vi "Main Page.vi"(8 "error in (no error)":errorcluster, 11 "Node Ptr":T1 format="%.0x") -> (0 "error out":errorcluster)   [LabVIEW 2015, in "Waveform-Processing-Custom-Device System Explorer.lvlib"]
uses:
  Waveform-Processing-Custom-Device System Explorer.lvlib
  <vilib>/NI Veristand/Custom Device API/Custom Device Item Ref.ctl
  Shared/Types/FG Action.ctl
  Types/UI Refs Ctl.ctl
  Shared/Constants.vi
  <vilib>/NI Veristand/Custom Device API/Set Item Property (Boolean).vi
  <vilib>/NI VeriStand/Custom Device API/Custom Device API.lvlib
  Shared/Waveform-Processing-Custom-Device Shared.lvlib
  Shared/Running Average/Running Average.lvlib
  Shared/Single Point/SinglePoint.lvlib
panel:
  in  "Header 2":cluster{"Section Name":string}={"Section Name"="Custom Device Item Settings"}
  out "Task Rate (Hz)":dbl
  in  "Buffer Length (s)":dbl format="%#_6f"
  out "Buffer Length (samples)":u32
  in  "Description":string
  in  "Remove Channel":bool
  in  "Add Channel":bool
  in  "Selected Waveforms":i32[](listbox)
  in  "Waveform Task":u16(ring) items=["Waveform1"=11, "Waveform2"=15]
  in  "Available Waveforms":i32[](listbox)
  in  "Single-point":bool
  in  "Running Average":bool
  in  "Header":cluster{"Section Name":string}={"Section Name"="Custom Device Item Settings"}
  in  "Name":string
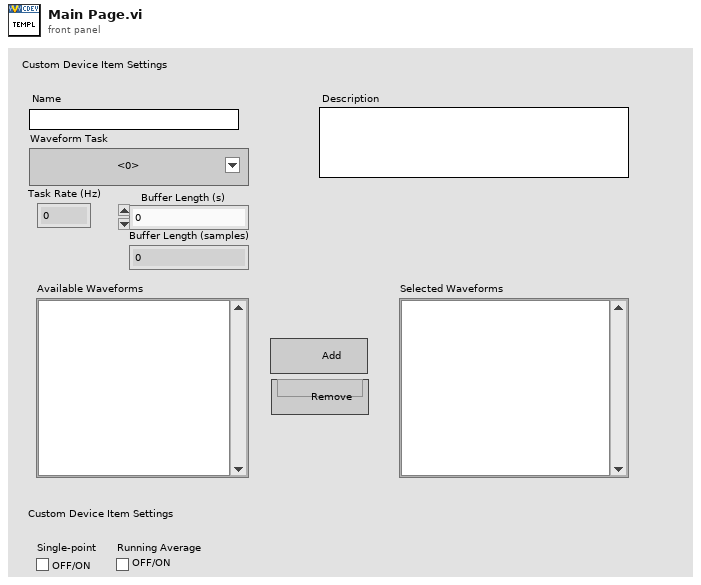
[diagram p1: front panel]
types:
  T1 = typedef "Custom Device API.lvlib/Custom Device Item Ref.ctl" = u64
  T2 = typedef "Waveform-Processing-Custom-Device Shared.lvlib/UI Refs Ctl.ctl" = cluster{"Selected Waveforms":refnum<vi>, "Available Waveforms":refnum<vi>, "Wfm Task Rate (Hz)":refnum<vi>, "Buffer Length (s)":refnum<vi>, "Buffer Length (samples)":refnum<vi>, "Add Channel":refnum<vi>, "Remove Channel":refnum<vi>, "Running Average":refnum<vi>, "Single-point":refnum<vi>, "Waveform Task":refnum<vi>}
  T3 = typedef "Waveform-Processing-Custom-Device Shared.lvlib/FG Action.ctl" = enum8{"GET", "SET"}
  T4 = typedef "Custom Device API.lvlib/Custom Device Item Info.ctl" = cluster{"Name":string, "Is Channel":bool, "GUID":string, "Is Waveform":bool}
  T5 = typedef "Waveform-Processing-Custom-Device Shared.lvlib/Custom Device Settings.ctl" = cluster{"CD Task Dependency":T1, "CD Task Dependency Ref":T1, "CD Task Available Wfms":string[], "CD Task Selected Wfms":string[], "Buffer Length (s)":dbl, "Buffer Length (samples)":u32, "Single-point Enabled":bool, "Running Average Enabled":bool, "Task Rate":dbl}
  T6 = typedef "Custom Device API.lvlib/Custom Device Commands.ctl" = enum16{"Default", "Item renamed", "Shutdown", "Dynamic button pressed"}
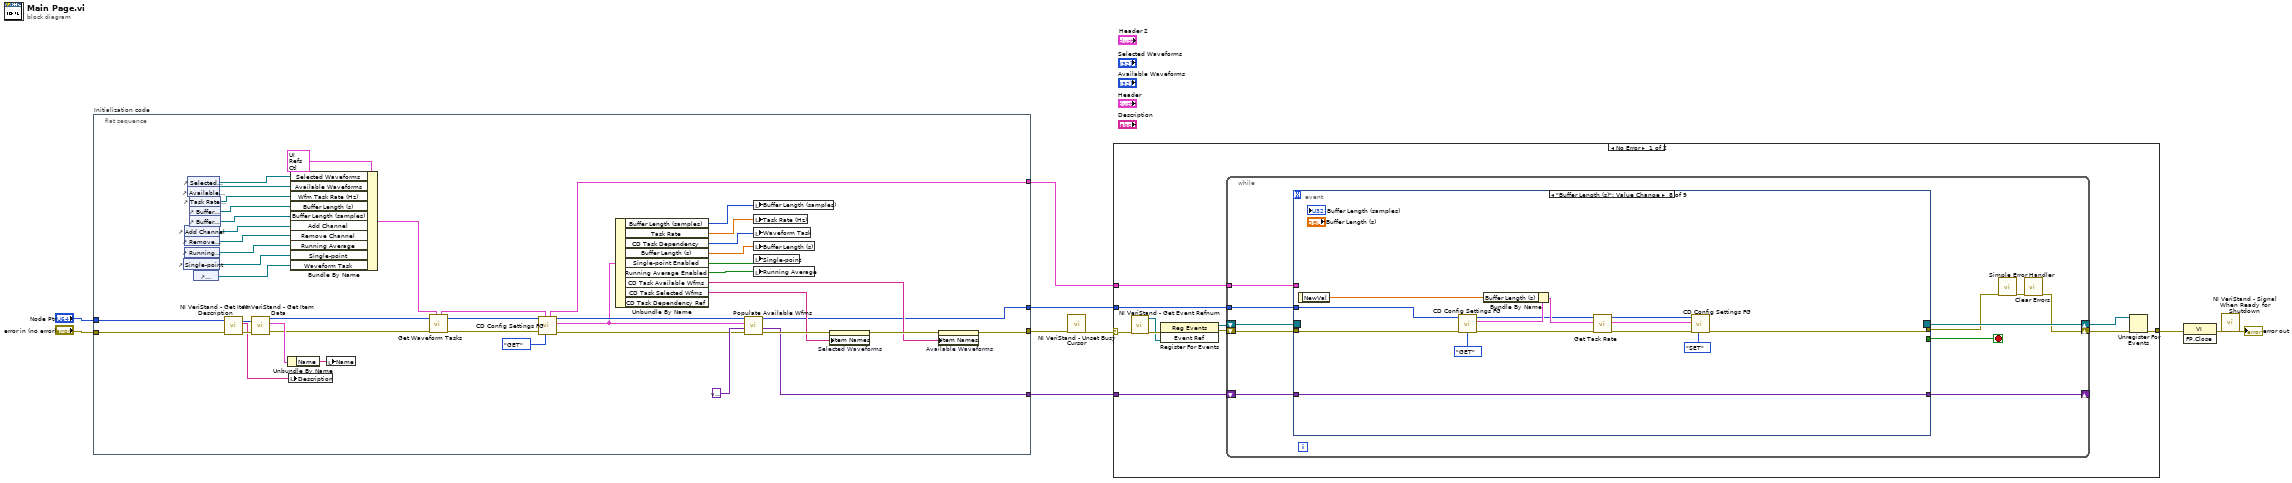
[diagram p0: block diagram]
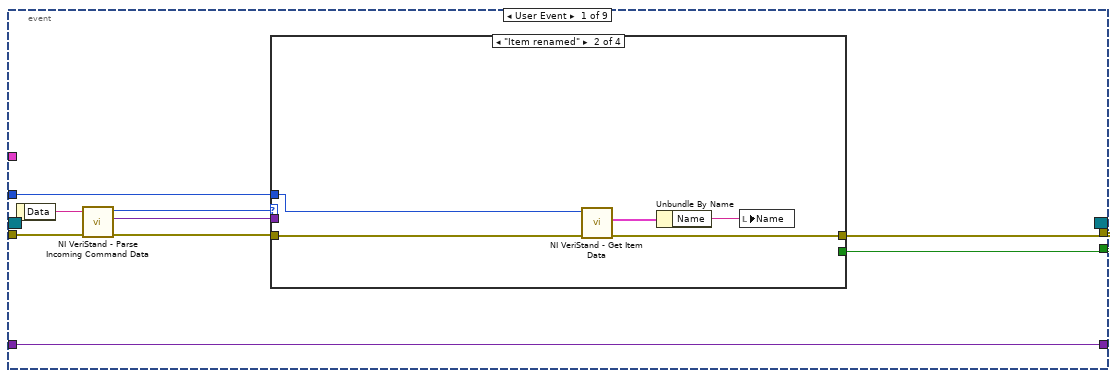
[diagram p2: hidden frame]
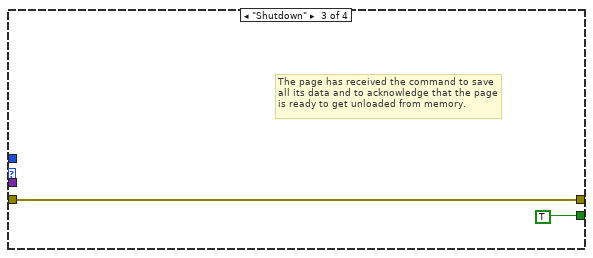
[diagram p4: hidden frame]
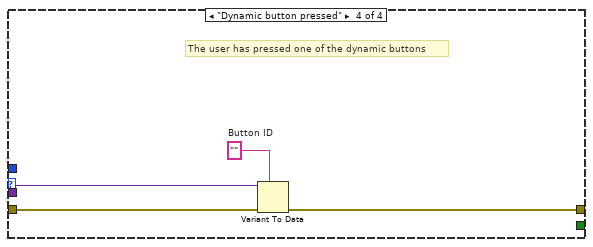
[diagram p5: hidden frame]
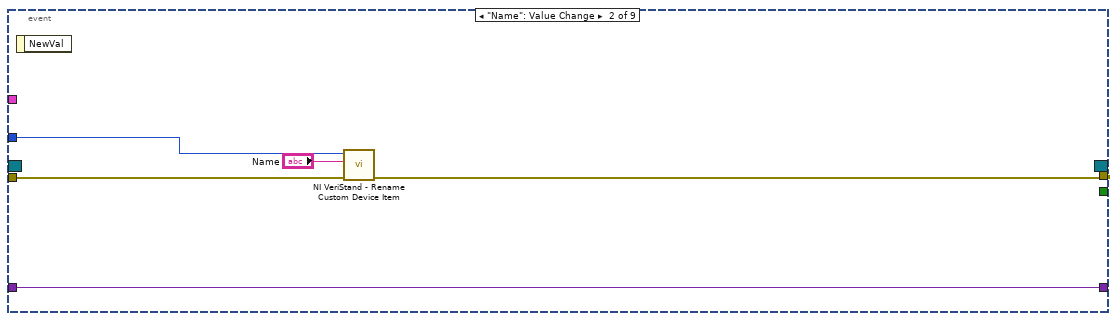
[diagram p6: hidden frame]
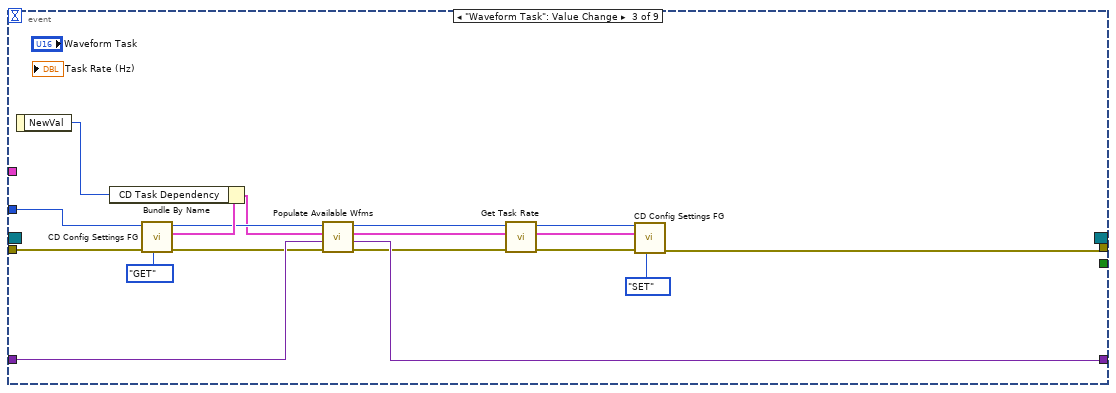
[diagram p7: hidden frame]
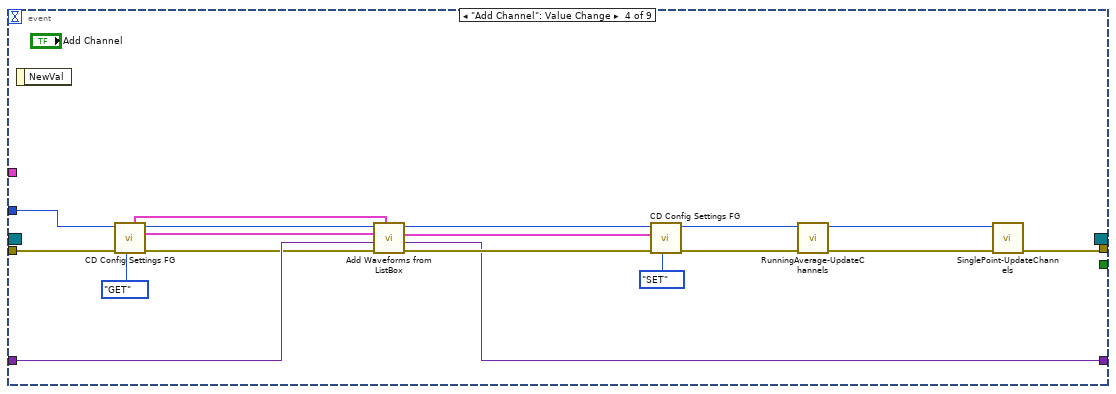
[diagram p8: hidden frame]
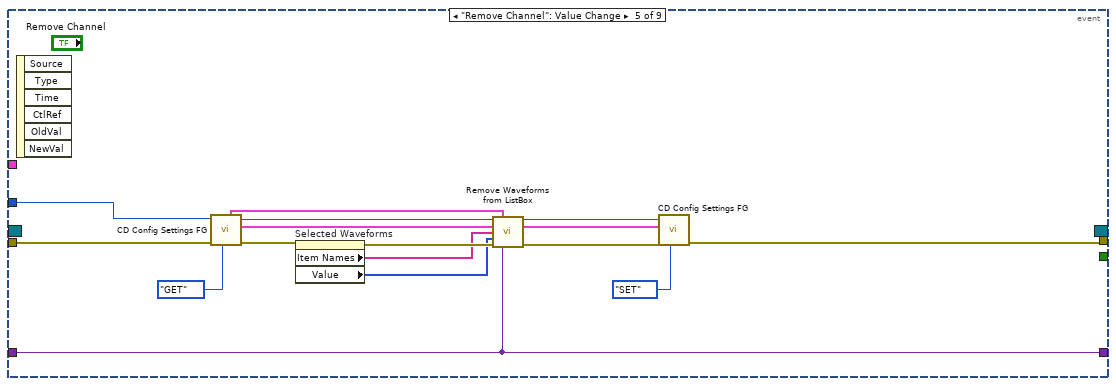
[diagram p9: hidden frame]
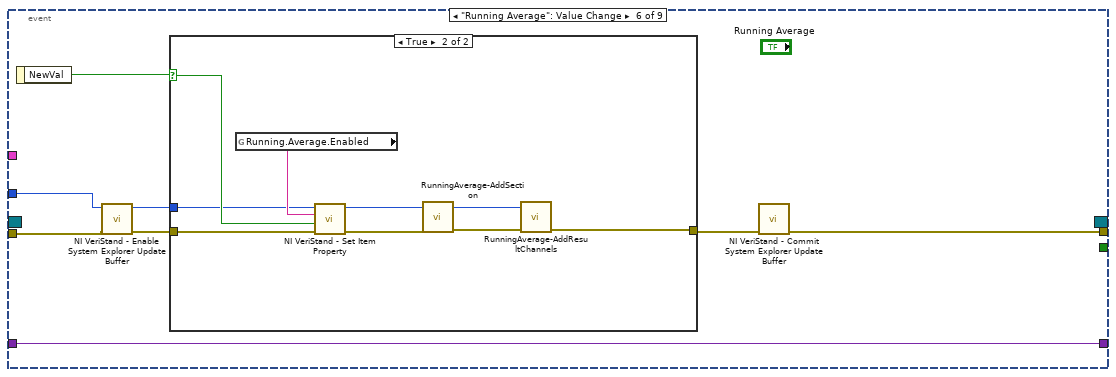
[diagram p10: hidden frame]
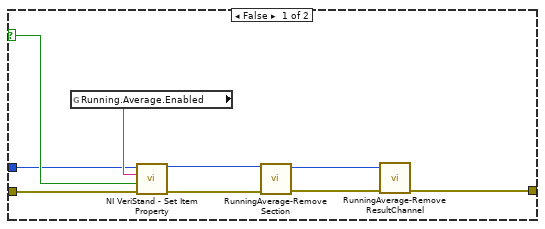
[diagram p11: hidden frame]
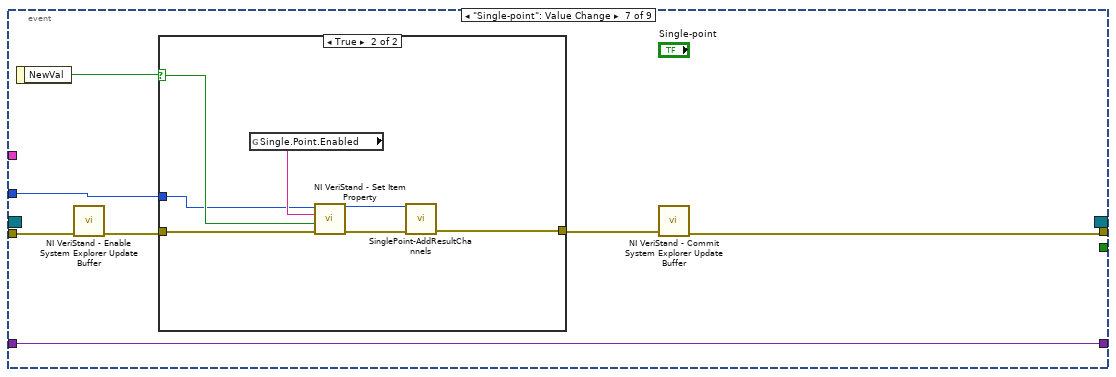
[diagram p12: hidden frame]
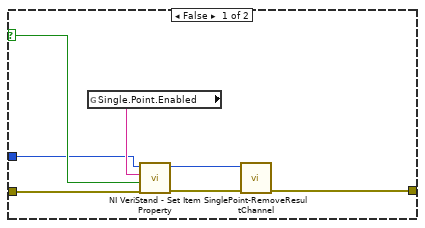
[diagram p13: hidden frame]
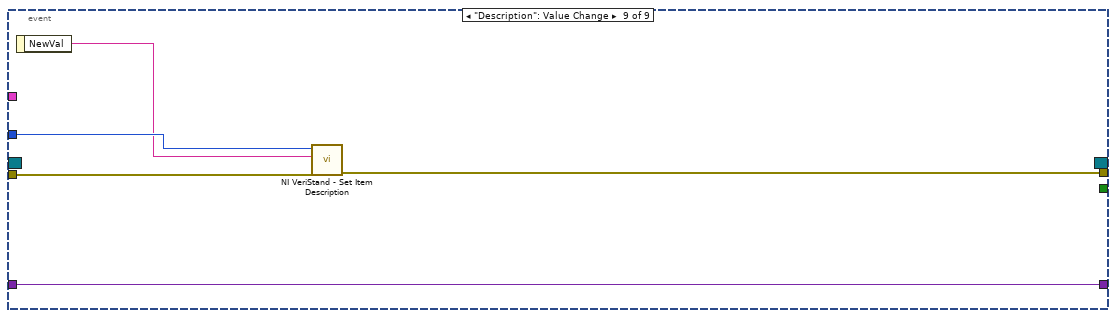
[diagram p14: hidden frame]
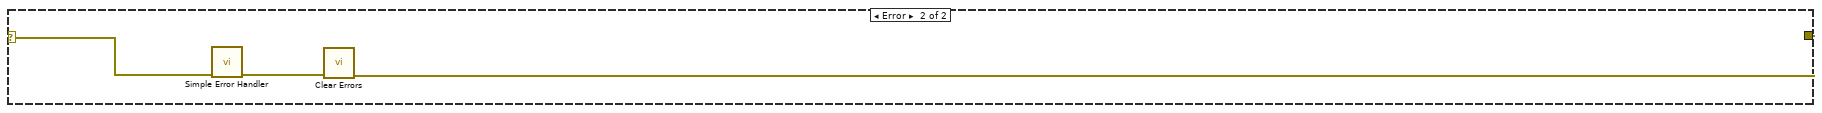
[diagram p15: hidden frame]
diagram:
  n1 = flat-sequence "Initialization code" {
    tunnel: "error in (no error)" -> [w52]
    tunnel: "Node Ptr" -> [w51]
    tunnel: [w38] -> w1
    tunnel: [w15] -> w4
    tunnel: [w13] -> w3
    tunnel: [w16] -> w2
    frame #0 {
      n2 = control-ref of="Single-point"() -> (w35:refnum<vi>)
      n3 = control-ref of="Add Channel"() -> (w32:refnum<vi>)
      n4 = control-ref of="Remove Channel"() -> (w33:refnum<vi>)
      n5 = control-ref of="Running Average"() -> (w34:refnum<vi>)
      n6 = control-ref of="Selected Waveforms"() -> (w27:refnum<vi>)
      n7 = control-ref of="Available Waveforms"() -> (w28:refnum<vi>)
      n8 = control-ref of="Task Rate (Hz)"() -> (w29:refnum<vi>)
      n9 = control-ref of="Buffer Length (s)"() -> (w30:refnum<vi>)
      n10 = control-ref of="Buffer Length (samples)"() -> (w31:refnum<vi>)
      n11 = control-ref of="Waveform Task"() -> (w17:refnum<vi>)
      n12 = call <vilib>:"NI VeriStand - Get Item Description.vi"("error in (no error)"=w52, "Item Ref in"=w51) -> ("error out"=w50:errorcluster, "Description"=w47:string, "Item Ref out"=w53:T1)  [unwired: 7 out]
      n13 = call <vilib>:"NI VeriStand - Get Item Data.vi"("error in (no error)"=w50, "Item Ref in"=w53) -> ("error out"=w24:errorcluster, "Item Info"=w49:T4, "Item Ref out"=w18:T1)  [unwired: 7 out]
      n14 = Unbundle By Name(w49) -> ("Name"=w48:string)
      n15 = local write "Description"(w47) -> ()
      n16 = Bundle By Name(cluster=T2 {"Selected Waveforms"=refnum, "Available Waveforms"=refnum, "Wfm Task Rate (Hz)"=refnum, "Buffer Length (s)"=refnum, "Buffer Length (samples)"=refnum, "Add Channel"=refnum, "Remove Channel"=refnum, "Running Average"=refnum, "Single-point"=refnum, "Waveform Task"=refnum} ("UI Refs"), "Selected Waveforms"=w27, "Available Waveforms"=w28, "Wfm Task Rate (Hz)"=w29, "Buffer Length (s)"=w30, "Buffer Length (samples)"=w31, "Add Channel"=w32, "Remove Channel"=w33, "Running Average"=w34, "Single-point"=w35, "Waveform Task"=w17) -> (w23:T2)
      n17 = local write "Name"(w48) -> ()
      n18 = call "Get Waveform Tasks.vi"("Custom Device ref in"=w18, "error in"=w24, "UI Refs in"=w23) -> ("UI Refs out"=w22:T2, "Custom Device ref out"=w21:T1, "error out"=w25:errorcluster)  [unwired: 5 in]
      n19 = call "CD Config Settings FG.vi"("Action"=FG_Action."GET", "UI Refs"=w22, "error in (no error)"=w25, "Item Ref"=w21) -> ("error out"=w20:errorcluster, "CD Settings out"=w11:T5, "Item Ref out"=w19:T1, "UI Refs out"=w16:T2)  [unwired: 4 in]
      n20 = Unbundle By Name(w11) -> ("Buffer Length (samples)"=w12:u32, "Task Rate"=w14:dbl, "CD Task Dependency"=w26:T1, "Buffer Length (s)"=w44:dbl, "Single-point Enabled"=w46:bool, "Running Average Enabled"=w45:bool, "CD Task Available Wfms"=w39:string[], "CD Task Selected Wfms"=w40:string[])  [unwired: 1 out]
      n21 = call "Populate Available Wfms.vi"("error in"=w20, "ListBox Variant"=variant, "CD Settings"=w11, "CustomDevice Ref"=w19) -> ("error out"=w42:errorcluster, "ListBox Variant"=w38:variant, "CustomDevice Ref"=w13:T1)  [unwired: 4 in, 1 out]
      n22 = local write "Buffer Length (samples)"(w12) -> ()
      n23 = local write "Task Rate (Hz)"(w14) -> ()
      n24 = local write "Waveform Task"(w26) -> ()
      n25 = local write "Buffer Length (s)"(w44) -> ()
      n26 = local write "Single-point"(w46) -> ()
      n27 = local write "Running Average"(w45) -> ()
      n28 = property on="Selected Waveforms" class="LstBox (strict)"(error in=w42, "Item Names"=w40) -> (error out=w41:errorcluster)  [unwired: 1 in, 1 out]
      n29 = property on="Available Waveforms" class="LstBox (strict)"(error in=w41, "Item Names"=w39) -> (error out=w15:errorcluster)  [unwired: 1 in, 1 out]
    }
  }
  n30 = call <vilib>:"NI VeriStand - Unset Busy Cursor.vi"("error in (no error)"=w4) -> ("error out"=w6:errorcluster)  [unwired: 10 out]
  n31 = case shown="No Error" w6 {
    selector: w6 -> [w57 w221]
    tunnel: [w61 w219] -> w10
    tunnel: w3 -> [w56 _]
    tunnel: w1 -> [w55 _]
    tunnel: w2 -> [w54 _]
    frame No Error {
      n32 = call <vilib>:"NI VeriStand - Get Event Refnum.vi"("error in (no error)"=w57) -> ("error out"=w64:errorcluster, "Event Ref"=w60:refnum<user-event>)  [unwired: 9 out]
      n33 = register-events(error in=w64, w60) -> (reference out=w58:refnum<event-registration>, error out=w59:errorcluster)  [unwired: 1 in]
      n34 = while {
        shift-right: [w71] -> w62
        shift-left: w59 -> [w67]
        shift-right: [w75] -> w63
        shift-left: w58 -> [w74]
        tunnel: w56 -> [w70]
        shift-right: [w69] -> _
        shift-left: w55 -> [w68]
        tunnel: w54 -> [w65]
        stop <- w73 stop-if-true
        n35 = event shown="[7] \"Buffer Length (s)\": Value Change" {
          selector: w74 -> [_ _ _ _ _ _ _ _ _]
          dyn-events: [_ _ _ _ _ _ _ _ _] -> w75
          timeout: _ -> [_ _ _ _ _ _ _ _ _]
          tunnel: w67 -> [w84 w101 w116 w131 w150 w157 w182 w212 w218]
          tunnel: [w80 _ _ _ _ _ _ _ _] -> w73
          tunnel: [w79 w100 w102 w126 w139 w154 w179 w200 w217] -> w66
          tunnel: w70 -> [w77 w98 w115 w137 w153 w159 w184 w210 w216]
          tunnel: [w76 w97 w119 w121 w138 w158 w183 w213 w214] -> w69
          tunnel: w68 -> [w76 w97 w118 w123 w138 w158 w183 w213 w214]
          tunnel: w65 -> [_ _ _ _ _ _ _ _ _]
          event User Event {
            n36 = event-data() -> ("Data"=w83:string)  [unwired: 1 out]
            n37 = call <vilib>:"NI VeriStand - Parse Incoming Command Data.vi"("error in (no error)"=w84, "Incoming data"=w83) -> ("error out"=w82:errorcluster, "Outgoing data"=w78:variant, "Action"=w81:T6)  [unwired: 7 out]
            n38 = case shown="\"Item renamed\"" w81 {
              tunnel: w82 -> [w85 w90 w91 w96]
              tunnel: [_ _ TRUE _] -> w80
              tunnel: [w85 w88 w91 w93] -> w79
              tunnel: w78 -> [_ _ _ w95]
              tunnel: w77 -> [_ w86 _ _]
              frame "Default", Default {
              }
              frame "Item renamed" {
                n39 = call <vilib>:"NI VeriStand - Get Item Data.vi"("error in (no error)"=w90, "Item Ref in"=w86) -> ("error out"=w88:errorcluster, "Item Info"=w89:T4)  [unwired: 8 out]
                n40 = Unbundle By Name(w89) -> ("Name"=w87:string)
                n41 = local write "Name"(w87) -> ()
              }
              frame "Shutdown" {
                # "The page has received the command to save all its data and to acknowledge that the page is ready to get unloaded from memory."
              }
              frame "Dynamic button pressed" {
                w94 = ""  # Button ID
                # "The user has pressed one of the dynamic buttons"
                n42 = Variant To Data(error in=w96, type=w94, Variant=w95) -> (error out=w93:errorcluster)  [unwired: 1 out]
              }
            }
          }
          event "Name": Value Change {
            n43 = event-data() -> ()  [unwired: 2 out]
            n44 = call <vilib>:"NI VeriStand - Rename Custom Device Item.vi"("error in (no error)"=w101, "New Name"="Name", "Item Ref in"=w98) -> ("error out"=w100:errorcluster)  [unwired: 1 in, 7 out]
          }
          event "Waveform Task": Value Change {
            n45 = event-data() -> ("NewVal"=w117:u16)  [unwired: 1 out]
            n46 = call "CD Config Settings FG.vi"("Action"=FG_Action."GET", "error in (no error)"=w116, "Item Ref"=w115) -> ("error out"=w111:errorcluster, "CD Settings out"=w114:T5, "Item Ref out"=w110:T1)  [unwired: 5 in, 1 out]
            n47 = Bundle By Name(cluster=w114, "CD Task Dependency"=w117) -> (w109:T5)
            n48 = call "Populate Available Wfms.vi"("error in"=w111, "ListBox Variant"=w118, "CD Settings"=w109, "CustomDevice Ref"=w110) -> ("error out"=w108:errorcluster, "ListBox Variant"=w119:variant, "CD Settings out"=w107:T5, "CustomDevice Ref"=w106:T1)  [unwired: 4 in]
            n49 = call "Get Task Rate.vi"("error in"=w108, "CD Settings"=w107, "CustomDevice Ref"=w106) -> ("error out"=w104:errorcluster, "CD Settings out"=w103:T5, "CustomDevice Ref out"=w105:T1)  [unwired: 6 in]
            n50 = call "CD Config Settings FG.vi"("Action"=FG_Action."SET", "error in (no error)"=w104, "CD Settings in"=w103, "Item Ref"=w105) -> ("error out"=w102:errorcluster)  [unwired: 4 in, 3 out]
          }
          event "Add Channel": Value Change {
            n51 = event-data() -> ()  [unwired: 2 out]
            n52 = call "CD Config Settings FG.vi"("Action"=FG_Action."GET", "error in (no error)"=w131, "Item Ref"=w137) -> ("error out"=w122:errorcluster, "CD Settings out"=w133:T5, "Item Ref out"=w130:T1, "UI Refs out"=w120:T2)  [unwired: 5 in]
            n53 = call "Add Waveforms from ListBox.vi"("UI Refs"=w120, "error in (no error)"=w122, "Wfm Ref LUT"=w123, "CD Settings in"=w133, "Custom Device Ref in"=w130) -> ("error out"=w136:errorcluster, "Wfm Ref LUT out"=w121:variant, "CD Settings out"=w132:T5, "Custom Device Ref out"=w129:T1)  [unwired: 1 in]
            n54 = call "CD Config Settings FG.vi"("Action"=FG_Action."SET", "error in (no error)"=w136, "CD Settings in"=w132, "Item Ref"=w129) -> ("error out"=w128:errorcluster, "Item Ref out"=w125:T1)  [unwired: 4 in, 2 out]
            n55 = call "RunningAverage-UpdateChannels.vi"("Error in"=w128, "Custom Device ref in"=w125) -> ("Error out"=w127:errorcluster, "Custom Device ref out"=w124:T1)  [unwired: 8 in]
            n56 = call "SinglePoint-UpdateChannels.vi"("Error in"=w127, "Custom Device ref in"=w124) -> ("Error out"=w126:errorcluster)  [unwired: 8 in, 1 out]
          }
          event "Remove Channel": Value Change {
            n57 = event-data() -> ()  [unwired: 7 out]
            n58 = call "CD Config Settings FG.vi"("Action"=FG_Action."GET", "error in (no error)"=w150, "Item Ref"=w153) -> ("error out"=w149:errorcluster, "CD Settings out"=w144:T5, "Item Ref out"=w143:T1, "UI Refs out"=w142:T2)  [unwired: 5 in]
            n59 = property on="Selected Waveforms" class="LstBox (strict)"(error in=w149) -> (error out=w148:errorcluster, "Item Names"=w145:string[], "Value"=w146:i32[])  [unwired: 1 in, 1 out]
            n60 = call "Remove Waveforms from ListBox.vi"("Custom Device Ref in"=w143, "UI Refs"=w142, "CD Settings in"=w144, "Item Names"=w145, "Value"=w146, "error in (no error)"=w148, "Waveform Ref LUT"=w138) -> ("Custom Device Ref out"=w141:T1, "CD Settings out"=w140:T5, "error out"=w147:errorcluster)  [unwired: 6 in]
            n61 = call "CD Config Settings FG.vi"("Action"=FG_Action."SET", "error in (no error)"=w147, "CD Settings in"=w140, "Item Ref"=w141) -> ("error out"=w139:errorcluster)  [unwired: 4 in, 3 out]
          }
          event "Running Average": Value Change {
            n62 = event-data() -> ("NewVal"=w160:bool)  [unwired: 1 out]
            n63 = call <vilib>:"NI VeriStand - Enable System Explorer Update Buffer.vi"("error in (no error)"=w157) -> ("error out"=w156:errorcluster)  [unwired: 10 in]
            n64 = case shown="True" w160 {
              selector: w160 -> [w167 w177]
              tunnel: w156 -> [w169 w170]
              tunnel: [w162 w171] -> w155
              tunnel: w159 -> [w166 w174]
              frame False {
                n65 = global read "Constants.vi" "Running.Average.Enabled"() -> (w168:string)
                n66 = call-poly <vilib>:"NI VeriStand - Set Item Property.vi"("error in (no error)"=w169, "Value"=w167, "Property Name"=w168, "Item Ref in"=w166) -> ("error out"=w164:errorcluster, "Item Ref out"=w165:T1)  [unwired: 5 in, 1 out]
                n67 = call "RunningAverage-RemoveSection.vi"("Error in"=w164, "Custom Device ref"=w165) -> ("Error out"=w163:errorcluster, "Custom Device ref out"=w161:T1)  [unwired: 8 in]
                n68 = call "RunningAverage-RemoveResultChannel.vi"("Error in"=w163, "Custom Device ref"=w161) -> ("Error out"=w162:errorcluster)  [unwired: 8 in, 1 out]
              }
              frame True {
                n69 = global read "Constants.vi" "Running.Average.Enabled"() -> (w178:string)
                n70 = call-poly <vilib>:"NI VeriStand - Set Item Property.vi"("error in (no error)"=w170, "Value"=w177, "Property Name"=w178, "Item Ref in"=w174) -> ("error out"=w176:errorcluster, "Item Ref out"=w175:T1)  [unwired: 5 in, 1 out]
                n71 = call "RunningAverage-AddSection.vi"("Error in"=w176, "Custom Device ref"=w175) -> ("Error out"=w173:errorcluster, "Custom Device ref out"=w172:T1)  [unwired: 8 in]
                n72 = call "RunningAverage-AddResultChannels.vi"("Error in"=w173, "Custom Device ref"=w172) -> ("Error out"=w171:errorcluster)  [unwired: 8 in, 1 out]
              }
            }
            n73 = call <vilib>:"NI VeriStand - Commit System Explorer Update Buffer.vi"("error in (no error)"=w155) -> ("error out"=w154:errorcluster)  [unwired: 10 in]
          }
          event "Single-point": Value Change {
            n74 = event-data() -> ("NewVal"=w185:bool)  [unwired: 1 out]
            n75 = call <vilib>:"NI VeriStand - Enable System Explorer Update Buffer.vi"("error in (no error)"=w182) -> ("error out"=w181:errorcluster)  [unwired: 10 in]
            n76 = case shown="True" w185 {
              selector: w185 -> [w191 w197]
              tunnel: w181 -> [w187 w198]
              tunnel: [w186 w194] -> w180
              tunnel: w184 -> [w188 w193]
              frame False {
                n77 = global read "Constants.vi" "Single.Point.Enabled"() -> (w192:string)
                n78 = call-poly <vilib>:"NI VeriStand - Set Item Property.vi"("error in (no error)"=w187, "Value"=w191, "Property Name"=w192, "Item Ref in"=w188) -> ("error out"=w190:errorcluster, "Item Ref out"=w189:T1)  [unwired: 5 in, 1 out]
                n79 = call "SinglePoint-RemoveResultChannel.vi"("Error in"=w190, "Custom Device ref"=w189) -> ("Error out"=w186:errorcluster)  [unwired: 8 in, 1 out]
              }
              frame True {
                n80 = global read "Constants.vi" "Single.Point.Enabled"() -> (w199:string)
                n81 = call-poly <vilib>:"NI VeriStand - Set Item Property.vi"("error in (no error)"=w198, "Value"=w197, "Property Name"=w199, "Item Ref in"=w193) -> ("error out"=w196:errorcluster, "Item Ref out"=w195:T1)  [unwired: 5 in, 1 out]
                n82 = call "SinglePoint-AddResultChannels.vi"("Error in"=w196, "Custom Device ref"=w195) -> ("Error out"=w194:errorcluster)  [unwired: 8 in, 1 out]
              }
            }
            n83 = call <vilib>:"NI VeriStand - Commit System Explorer Update Buffer.vi"("error in (no error)"=w180) -> ("error out"=w179:errorcluster)  [unwired: 10 in]
          }
          event "Buffer Length (s)": Value Change {
            n84 = event-data() -> ("NewVal"=w208:dbl)  [unwired: 1 out]
            n85 = call "CD Config Settings FG.vi"("Action"=FG_Action."GET", "error in (no error)"=w212, "Item Ref"=w210) -> ("error out"=w206:errorcluster, "CD Settings out"=w209:T5, "Item Ref out"=w205:T1)  [unwired: 5 in, 1 out]
            n86 = Bundle By Name(cluster=w209, "Buffer Length (s)"=w208) -> (w207:T5)
            n87 = call "Get Task Rate.vi"("error in"=w206, "CD Settings"=w207, "CustomDevice Ref"=w205) -> ("error out"=w204:errorcluster, "CD Settings out"=w202:T5, "CustomDevice Ref out"=w203:T1)  [unwired: 6 in]
            n88 = call "CD Config Settings FG.vi"("Action"=FG_Action."SET", "error in (no error)"=w204, "CD Settings in"=w202, "Item Ref"=w203) -> ("error out"=w200:errorcluster)  [unwired: 4 in, 3 out]
          }
          event "Description": Value Change {
            n89 = event-data() -> ("NewVal"=w215:string)  [unwired: 1 out]
            n90 = call <vilib>:"NI VeriStand - Set Item Description.vi"("error in (no error)"=w218, "Description"=w215, "Item Ref in"=w216) -> ("error out"=w217:errorcluster)  [unwired: 8 out]
          }
        }
        n91 = call <vilib>:"Simple Error Handler.vi"("error in (no error)"=w66) -> ("error out"=w72:errorcluster)  [unwired: 1 in, 7 out]
        n92 = call <vilib>:"Clear Errors.vi"("error in (no error)"=w72) -> ("error out"=w71:errorcluster)  [unwired: 1 in, 5 out]
      }
      n93 = Unregister For Events(event registration refnum=w63, error in=w62) -> (error out=w61:errorcluster)
    }
    frame Error {
      n94 = call <vilib>:"Simple Error Handler.vi"("error in (no error)"=w221) -> ("error out"=w220:errorcluster)  [unwired: 1 in, 7 out]
      n95 = call <vilib>:"Clear Errors.vi"("error in (no error)"=w220) -> ("error out"=w219:errorcluster)  [unwired: 1 in, 5 out]
    }
  }
  n96 = invoke class="VI" method="FP.Close"(error in=w10) -> (error out=w9:errorcluster)  [unwired: 2 in, 2 out]
  n97 = call <vilib>:"NI VeriStand - Signal When Ready for Shutdown.vi"("error in (no error)"=w9) -> ("error out"=→"error out":errorcluster)  [unwired: 10 out]
